vi "get_image_size.vi"() -> ()   [LabVIEW 2010]
panel:
  in  "DEC size":dbl
  in  "RA size":dbl
  out "Cropped":sgl[][](array[numeric])
  in  "Astrometry":T1
  in  "ImgData":sgl[][](array[numeric])
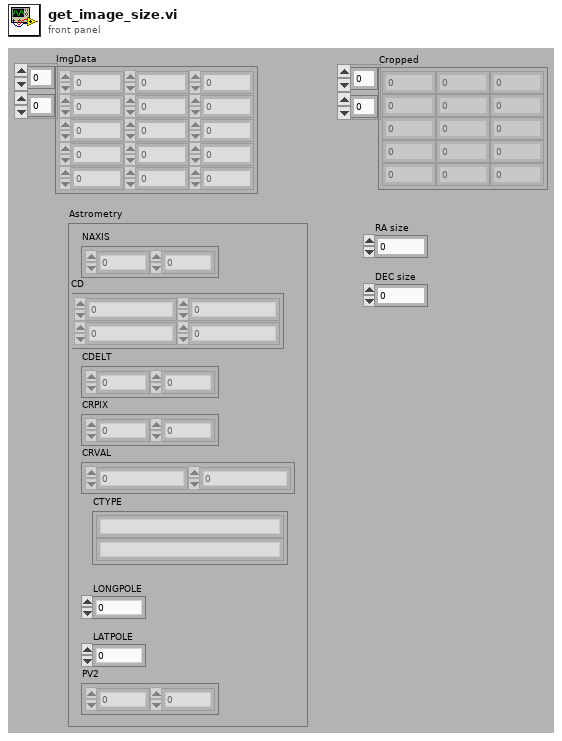
[diagram p1: front panel]
types:
  T1 = cluster{"NAXIS":dbl[], "CD":dbl[][], "CDELT":dbl[], "CRPIX":dbl[], "CTYPE":string[], "CRVAL":dbl[], "LONGPOLE":dbl, "LATPOLE":dbl, "PV2":dbl[]}
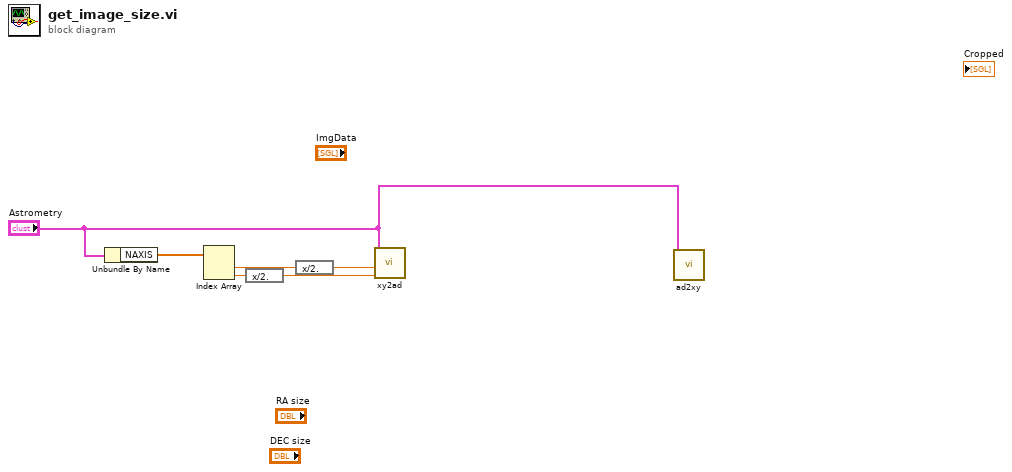
[diagram p0: block diagram]
diagram:
  n1 = Unbundle By Name("Astrometry") -> ("NAXIS"=w6:dbl[])
  n2 = Index Array(array=w6) -> (element #1=w5:dbl, element #2=w4:dbl)  [unwired: 2 in]
  n3 = expression code="x/2."(w4) -> (w2:dbl)
  n4 = expression code="x/2."(w5) -> (w3:dbl)
  n5 = call "xy2ad.vi"("Y (px)"=w2, "X (px)"=w3, "Astrometry"="Astrometry") -> ()  [unwired: 6 in, 3 out]
  n6 = call "ad2xy.vi"("Astrometry"="Astrometry") -> ()  [unwired: 8 in, 3 out]
